vi "Gamma_range.vi"(1 "Illuminant Table":string[][](array[string]), 2 "NumberOfRows":dbl) -> (0 "GammaInterval":dbl[](array[numeric]))   [LabVIEW 2014]
panel:
  out "LowestGamma":dbl
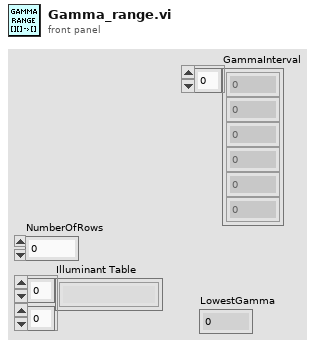
[diagram p1: front panel]
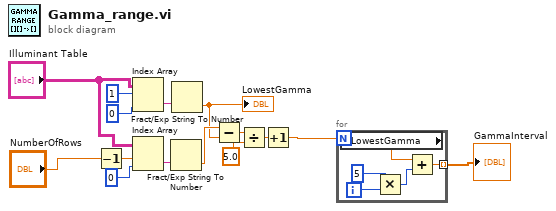
[diagram p0: block diagram]
diagram:
  n1 = Decrement(x="NumberOfRows") -> (x-1=w14:dbl)
  n2 = Index Array(array="Illuminant Table", index (row)=1, index (col)=0) -> (element=w11:string)
  n3 = Index Array(array="Illuminant Table", index (row)=w14, index (col)=0 ("disabled index (col)")) -> (element=w10:string)
  n4 = Fract/Exp String To Number(string=w10) -> (number=w9:dbl)  [unwired: 3 in, 1 out]
  n5 = Fract/Exp String To Number(string=w11) -> (number=w8:dbl)  [unwired: 3 in, 1 out]
  "LowestGamma" <- w8
  n6 = Subtract(x=w9, y=w8) -> (x-y=w7:dbl)
  n7 = Divide(x=w7, y=5.0) -> (x/y=w5:dbl)
  n8 = Increment(x=w5) -> (x+1=w2:dbl)
  n9 = for {
    N: w2 -> [_]
    tunnel: [w16] -> w1 mode=indexing
    i -> [w18]
    n10 = local read "LowestGamma"() -> (w19:dbl)
    n11 = Multiply(x=5, y=w18) -> (x*y=w20:i32)
    n12 = Add(x=w19, y=w20) -> (x+y=w16:dbl)
  }
  "GammaInterval" <- w1
